vi "RT-FPGA9229.vi"(0 "FPGA VI引用输入":refnum<k20> caption="FPGA VI引用输出", 5 "9229采样率":u32=32000, 7 "9229采样点数":u32=32000, 11 "错误输入":errorcluster) -> (3 "9229电压波形":waveform(sgl)[](array[waveform]), 4 "FPGA VI引用输出":refnum<k20>, 6 "9229数据":sgl[](array[numeric]), 8 "9229t0":timestamp, 10 "9229dt":dbl, 12 "9229剩余元素":u32, 13 "9229buff overflower":bool, 14 "9229buff underflower":bool, 15 "错误输出":errorcluster)   [LabVIEW 2013]
uses:
  <vilib>/rvi/interface/common/niFpgaWaitOnOcc.vi
  <vilib>/Utility/error.llb/Error Cluster From Error Code.vi
  <vilib>/rvi/errors/niLvFpgaAdjustHostInterfaceError.vi
  <vilib>/rvi/interface/nirviMethod/nirviMethod.xnode
  <vilib>/rvi/interface/nirviReadWriteControl/nirviReadWriteControl.xnode
  <vilib>/FPGAPlugInAG/Dynamic/niLvFpga_ReadFifo_Dynamic.vi
  <vilib>/rvi/errors/niLvFpgaMergeErrorWithErrorCode.vi
  NiFpgaLv.dll
  <vilib>/rvi/interface/Simulation/niFpgaSimulationCallBeginRW.vi
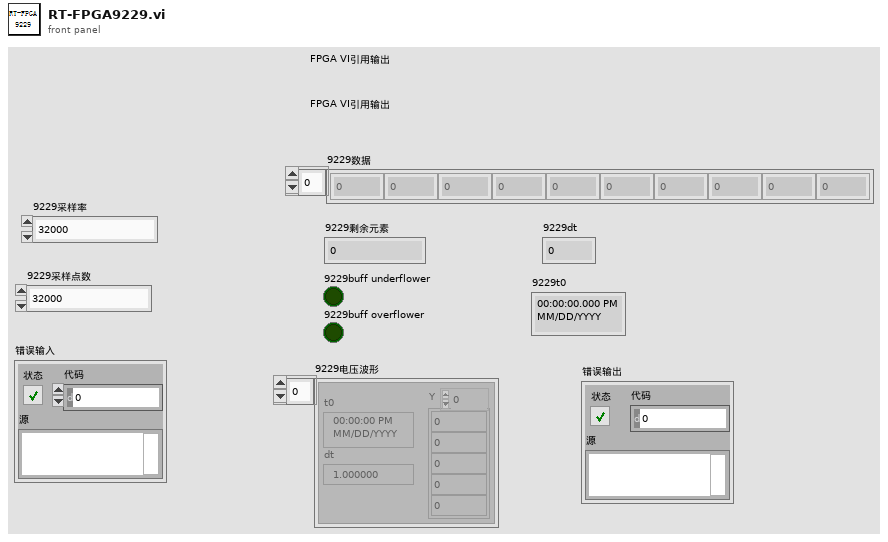
[diagram p1: front panel]
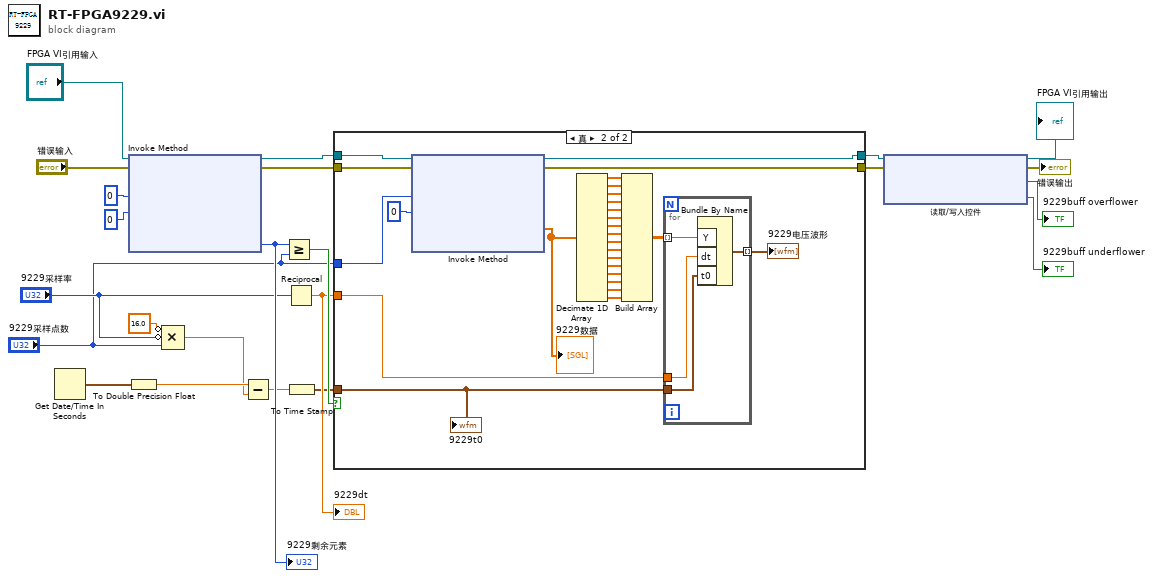
[diagram p0: block diagram]
diagram:
  n1 = Get Date/Time In Seconds() -> (seconds since 1Jan1904=w11:timestamp)
  n2 = xnode "Invoke Method"("FPGA VI引用输入"="FPGA VI引用输入", "错误输入"="错误输入", "元素数量"=u32 0, "超时(ms)"=0) -> ("FPGA VI引用输出"=w19:refnum<k20>, "错误输出"=w18:errorcluster, "剩余元素"=w21:u32)  [unwired: 1 out]
  "9229剩余元素" <- w21
  n3 = To Double Precision Float(number=w11) -> (double precision float=w10:dbl)
  n4 = Compound Arithmetic op=MULTIPLY(invert 16.0 ("值"), invert "9229采样率", "9229采样点数") -> (w9:dbl)
  n5 = Subtract(x=w10, y=w9) -> (x-y=w8:dbl)
  n6 = Greater Or Equal?(x=w21, y="9229采样点数") -> (x >= y?=w20:bool)
  n7 = Reciprocal(x="9229采样率") -> (1/x=w5:dbl)
  "9229dt" <- w5
  n8 = To Time Stamp(1:w8) -> (0:w4:timestamp)
  n9 = case shown="真" w20 {
    tunnel: w19 -> [w25 w52]
    tunnel: w18 -> [w24 w51]
    tunnel: "9229采样点数" -> [_ w50]
    tunnel: [w25 w48] -> w17
    tunnel: [w24 w47] -> w16
    tunnel: w5 -> [_ w28]
    tunnel: w4 -> [_ w27]
    frame False {
    }
    frame True {
      n10 = xnode "Invoke Method"("FPGA VI引用输入"=w52, "错误输入"=w51, "元素数量"=w50, "超时(ms)"=0) -> ("FPGA VI引用输出"=w48:refnum<k20>, "错误输出"=w47:errorcluster, "数据"=w30:sgl[])  [unwired: 1 out]
      "9229数据" <- w30
      n11 = Decimate 1D Array(w30) -> (w46:sgl[], w45:sgl[], w44:sgl[], w43:sgl[], w42:sgl[], w41:sgl[], w40:sgl[], w39:sgl[], w38:sgl[], w37:sgl[], w36:sgl[], w35:sgl[], w34:sgl[], w33:sgl[], w32:sgl[], w31:sgl[])
      n12 = Build Array(w46, w45, w44, w43, w42, w41, w40, w39, w38, w37, w36, w35, w34, w33, w32, w31) -> (w29:sgl[][])
      n13 = for {
        tunnel: w29 -> [w56] mode=indexing
        tunnel: w28 -> [w55]
        tunnel: w27 -> [w54]
        tunnel: [w53] -> w26 mode=indexing
        n14 = Bundle By Name("Y"=w56, "dt"=w55, "t0"=w54) -> (w53:waveform(sgl))  [unwired: 1 in]
      }
      "9229电压波形" <- w26
      "9229t0" <- w27
    }
  }
  n15 = xnode "读取/写入控件"("FPGA VI引用输入"=w17, "错误输入"=w16) -> ("FPGA VI引用输出"=→"FPGA VI引用输出":refnum<k20>, "错误输出"=→"错误输出":errorcluster, "9229buff overflower"=→"9229buff overflower":bool, "9229buff underflower"=→"9229buff underflower":bool)
